vi "MGI Number to Digits.vi"(0 "Number":i32, 1 "Base (10)":i32=10 min=2) -> (2 "Digits[]":i32[](array[numeric]))   [LabVIEW 2020]
doc: "Converts a single I32 into an array of digits, in order of increasing significance. If the input number is negative, the most significant digit (last element of the array) is also negative. All other digits are always non-negative. By default, the output digits are the digits used to represent the number in base 10, though the base can be changed. For example, the binary representation can be obtained by wiring the value 2 to the Base input. Note that Base is coerced to a minimum value of 2.\n\nAs long as no coersion is required, the original number can be recreated as\nN = Digits[0] * Base^0 + Digits[1] * Base^1 + Digits[2] * Base^2 + ... + Digits[n] * Base^n\n\nAuthored by Thomas Henage\nsupport@mooregoodideas.com\nwww.mooregoodideas.com\n\nCopyright (c) 2010, Moore Good Ideas, Inc.\n\nAll rights reserved.\n\nRedistribution and use in source and binary forms, with or without modification, are permitted provided that the following conditions are met:\n\n * Redistributions of source code must retain the above copyright notice, this list of conditions and the following disclaimer.\n * Redistributions in binary form must reproduce the above copyright notice, this list of conditions and the following disclaimer in the documentation and/or other materials provided with the distribution.\n * Neither the name of Moore Good Ideas, Inc. nor the names of its contributors may be used to endorse or promote products derived from this software without specific prior written permission.\n\nTHIS SOFTWARE IS PROVIDED BY THE COPYRIGHT HOLDERS AND CONTRIBUTORS \"AS IS\" AND ANY EXPRESS OR IMPLIED WARRANTIES, INCLUDING, BUT NOT LIMITED TO, THE IMPLIED WARRANTIES OF MERCHANTABILITY AND FITNESS FOR A PARTICULAR PURPOSE ARE DISCLAIMED. IN NO EVENT SHALL THE COPYRIGHT OWNER OR CONTRIBUTORS BE LIABLE FOR ANY DIRECT, INDIRECT, INCIDENTAL, SPECIAL, EXEMPLARY, OR CONSEQUENTIAL DAMAGES (INCLUDING, BUT NOT LIMITED TO, PROCUREMENT OF SUBSTITUTE GOODS OR SERVICES; LOSS OF USE, DATA, OR PROFITS; OR BUSINESS INTERRUPTION) HOWEVER CAUSED AND ON ANY THEORY OF LIABILITY, WHETHER IN CONTRACT, STRICT LIABILITY, OR TORT (INCLUDING NEGLIGENCE OR OTHERWISE) ARISING IN ANY WAY OUT OF THE USE OF THIS SOFTWARE, EVEN IF ADVISED OF THE POSSIBILITY OF SUCH DAMAGE."
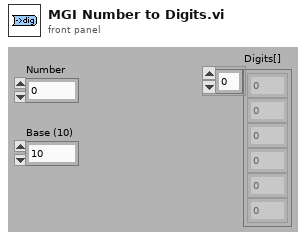
[diagram p1: front panel]
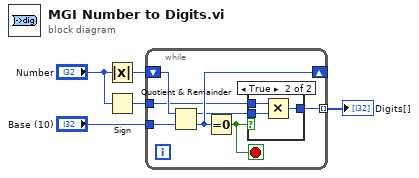
[diagram p0: block diagram]
diagram:
  n1 = Absolute Value(x="Number") -> (abs(x)=w4:i32)
  n2 = Sign(1:"Number") -> (0:w2:i32)
  n3 = while {
    tunnel: "Base (10)" -> [w12]
    tunnel: [w7] -> w5 mode=indexing
    shift-right: [w10] -> _
    shift-left: w4 -> [w11]
    tunnel: w2 -> [w6]
    stop <- w8 stop-if-true
    n4 = Quotient & Remainder(x=w11, y=w12) -> (x-y*floor(x/y)=w9:i32, floor(x/y)=w10:i32)
    n5 = Equal To 0?(x=w10) -> (x = 0?=w8:bool)
    n6 = case shown="True" w8 {
      tunnel: w9 -> [w13 w16]
      tunnel: [w13 w15] -> w7
      tunnel: w6 -> [_ w14]
      frame False {
      }
      frame True {
        n7 = Multiply(x=w14, y=w16) -> (x*y=w15:i32)
      }
    }
  }
  "Digits[]" <- w5
